vi "CAN_initialize.vi"() -> (0 "Array 2":errorcluster[](array[cluster]), 1 "Array":refnum<class "sbCANopenBaseClass.lvclass">[](array[class]), 2 "Motors to use":bool[](array[boolean]))   [LabVIEW 2017]
uses:
  <vilib>/addons/Maxon Motor/EPOS2 CANopen/CANopen/sbCANopenBaseClass.lvclass
  <vilib>/addons/Maxon Motor/EPOS2 CANopen/EPOS2 Support Files/Typedefs/EPOS2 Config Data Input Current.ctl
  <vilib>/addons/Maxon Motor/EPOS2 CANopen/EPOS2 Support Files/Typedefs/EPOS2 Velocity Units.ctl
  <vilib>/addons/Maxon Motor/EPOS2 CANopen/EPOS2 Support Files/Polymorphic SubVIs/Config/EPOS2 Current Mode Configure.vi
  <vilib>/imath/engines/lvmath2/RunTimeEngine/BuiltInFunctions/length/NIMS_length(GV).vi
  <instcachedir>/0/NIMS_length(GV)_08A3D13377FD4E4B96F5795FBF3698FA.lvgen/NIMS_length(GV)_08A3D13377FD4E4B96F5795FBF3698FA_003.vi
  <vilib>/imath/engines/lvmath2/RunTimeEngine/RangeToken/NIMS_Range_R2 - Integer.vi
  <instcachedir>/0/NIMS_Range_R2 - Integer_B2C3C6B11D0E4F789E1772ACB483EB02.lvgen/NIMS_Range_R2 - Integer_B2C3C6B11D0E4F789E1772ACB483EB02_000.vi
  <vilib>/imath/engines/lvmath2/RunTimeEngine/CommandStatement/MC_CommandStatement_break.vi
  <vilib>/imath/engines/lvmath2/RunTimeEngine/IndexRead/NIMS V(S).vi
  <instcachedir>/0/NIMS V(S)_0488751826AF41519A22953C041130DC.lvgen/NIMS V(S)_0488751826AF41519A22953C041130DC_003.vi
  <vilib>/imathl/engines/lvmath/Functions/Error Handling/Create Error.vi
  <vilib>/imath/engines/lvmath2/RunTimeEngine/VariableToken/NIMS_VariableToken_CondDefinedDefinedByReplace.vi
  <instcachedir>/0/NIMS_VariableToken_CondDefinedDefinedByReplace_D162CFFC24174562A9FEA619A91E1A56.lvgen/NIMS_VariableToken_CondDefinedDefinedByReplace_D162CFFC24174562A9FEA619A91E1A56_003.vi
  <vilib>/imath/engines/lvmath2/RunTimeEngine/IndexReplace/NIMS V(S)=S.vi
  <instcachedir>/0/NIMS V(S)=S_3F4D177D41884A9C969E5FA0B22E4B28.lvgen/NIMS V(S)=S_3F4D177D41884A9C969E5FA0B22E4B28_003.vi
  <vilib>/imath/engines/lvmath2/RunTimeEngine/VariableToken/NIMS_VariableToken_CondDefined.vi
  <instcachedir>/0/NIMS_VariableToken_CondDefined_6E7F1EE7F80E48298C84CF05BD736261.lvgen/NIMS_VariableToken_CondDefined_6E7F1EE7F80E48298C84CF05BD736261_004.vi
  <vilib>/imath/engines/lvmath2/RunTimeEngine/NodeEndStatement/NIMS_NodeEndStatement_Output.vi
  <instcachedir>/0/NIMS_NodeEndStatement_Output_53EC0D466D134D7ABD903AC30B43404B.lvgen/NIMS_NodeEndStatement_Output_53EC0D466D134D7ABD903AC30B43404B_004.vi
  <vilib>/imath/engines/lvmath2/RunTimeEngine/ErrorHandling/NIMS_Finalize Error.vi
  <vilib>/addons/Maxon Motor/EPOS2 CANopen/EPOS2 Library.lvlib
  <vilib>/addons/Maxon Motor/EPOS2 CANopen/CANopen/CANopen IndCom Interface/sdCANopenIndCom.lvclass
panel:
  out "size(s)":i32
  out "size(s) 2":i32
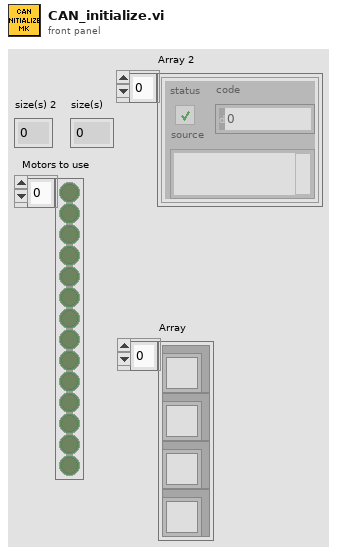
[diagram p1: front panel]
types:
  T1 = typedef "EPOS2 Library.lvlib/EPOS2 Config Data Input Current.ctl" = cluster{"Velocity Units":T2, "Max Velocity":i32}
  T2 = typedef "EPOS2 Library.lvlib/EPOS2 Velocity Units.ctl" = i8
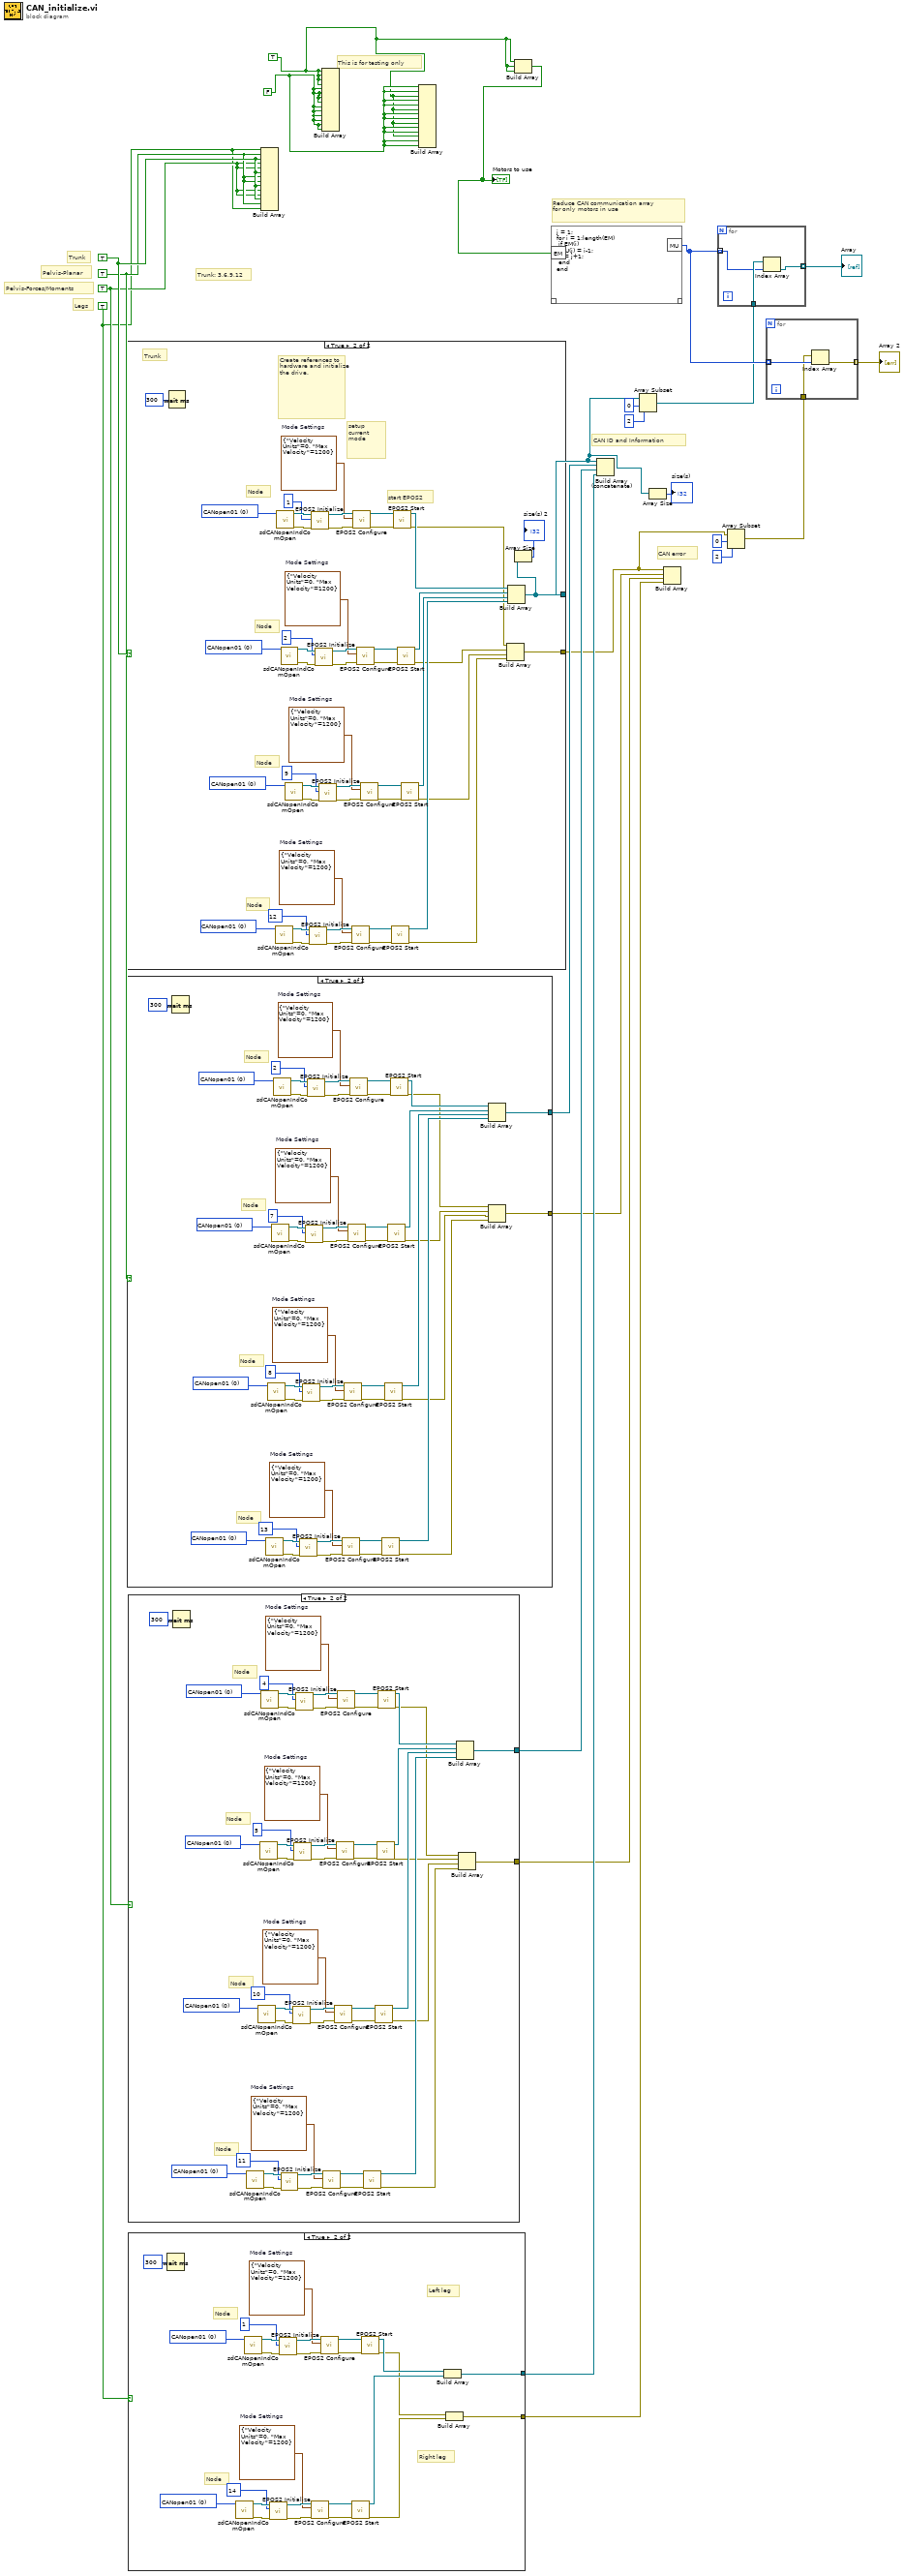
[diagram p0: block diagram]
diagram:
  w12 = FALSE
  w6 = TRUE
  w22 = TRUE
  w23 = TRUE
  w24 = TRUE
  w25 = TRUE
  # "This is for testing only"
  # "Trunk: 3,6,9,12"
  # "CAN error"
  # "CAN ID and Information"
  # "Reduce CAN communication array \nfor only motors in use"
  # "Legs"
  # "Pelvis-Forces/Moments"
  # "Pelvis-Planar"
  # "Trunk"
  n1 = case shown="True" w25 {
    tunnel: [_ w32] -> w11
    tunnel: [_ w33] -> w3
    frame False {
    }
    frame True {
      w43 = u32 0 items=["CANopen01", "CANopen02", "CANopen03", "CANopen04", "CANopen05", "CANopen06", "CANopen07", "CANopen08", "CANopen09", "CANopen10", "CANopen11", "CANopen12", "CANopen13", "CANopen14", "CANopen15", "CANopen16", "CANopen17", "CANopen18", "CANopen19", "CANopen20", "CANopen21", "CANopen22", "CANopen23", "CANopen24", "CANopen25", "CANopen26", "CANopen27", "CANopen28", "CANopen29", "CANopen30", "CANopen31", "CANopen32"] ("Interface Name")
      w44 = T1 {"Velocity Units"=0, "Max Velocity"=1200}  # Mode Settings
      w51 = u32 0 items=["CANopen01", "CANopen02", "CANopen03", "CANopen04", "CANopen05", "CANopen06", "CANopen07", "CANopen08", "CANopen09", "CANopen10", "CANopen11", "CANopen12", "CANopen13", "CANopen14", "CANopen15", "CANopen16", "CANopen17", "CANopen18", "CANopen19", "CANopen20", "CANopen21", "CANopen22", "CANopen23", "CANopen24", "CANopen25", "CANopen26", "CANopen27", "CANopen28", "CANopen29", "CANopen30", "CANopen31", "CANopen32"] ("Interface Name")
      w52 = T1 {"Velocity Units"=0, "Max Velocity"=1200}  # Mode Settings
      w59 = u32 0 items=["CANopen01", "CANopen02", "CANopen03", "CANopen04", "CANopen05", "CANopen06", "CANopen07", "CANopen08", "CANopen09", "CANopen10", "CANopen11", "CANopen12", "CANopen13", "CANopen14", "CANopen15", "CANopen16", "CANopen17", "CANopen18", "CANopen19", "CANopen20", "CANopen21", "CANopen22", "CANopen23", "CANopen24", "CANopen25", "CANopen26", "CANopen27", "CANopen28", "CANopen29", "CANopen30", "CANopen31", "CANopen32"] ("Interface Name")
      w60 = T1 {"Velocity Units"=0, "Max Velocity"=1200}  # Mode Settings
      w67 = u32 0 items=["CANopen01", "CANopen02", "CANopen03", "CANopen04", "CANopen05", "CANopen06", "CANopen07", "CANopen08", "CANopen09", "CANopen10", "CANopen11", "CANopen12", "CANopen13", "CANopen14", "CANopen15", "CANopen16", "CANopen17", "CANopen18", "CANopen19", "CANopen20", "CANopen21", "CANopen22", "CANopen23", "CANopen24", "CANopen25", "CANopen26", "CANopen27", "CANopen28", "CANopen29", "CANopen30", "CANopen31", "CANopen32"] ("Interface Name")
      w68 = T1 {"Velocity Units"=0, "Max Velocity"=1200}  # Mode Settings
      # "Node"
      # "Node"
      # "Node"
      # "Node"
      # "Trunk"
      # "Create references to hardware and initialize the drive."
      # "start EPOS2"
      # "setup current mode"
      n2 = Wait (ms)(milliseconds to wait=u32 300) -> ()  [unwired: 1 out]
      n3 = call <vilib>:"sdCANopenIndComOpen.vi"("Interface Name"=w43) -> ("error out"=w48:errorcluster, "SD CANopen Comm out"=w42:refnum<class "sbCANopenBaseClass.lvclass">)  [unwired: 9 in]
      n4 = call <vilib>:"sdCANopenIndComOpen.vi"("Interface Name"=w67) -> ("error out"=w72:errorcluster, "SD CANopen Comm out"=w66:refnum<class "sbCANopenBaseClass.lvclass">)  [unwired: 9 in]
      n5 = call <vilib>:"sdCANopenIndComOpen.vi"("Interface Name"=w59) -> ("error out"=w64:errorcluster, "SD CANopen Comm out"=w58:refnum<class "sbCANopenBaseClass.lvclass">)  [unwired: 9 in]
      n6 = call <vilib>:"sdCANopenIndComOpen.vi"("Interface Name"=w51) -> ("error out"=w56:errorcluster, "SD CANopen Comm out"=w50:refnum<class "sbCANopenBaseClass.lvclass">)  [unwired: 9 in]
      n7 = call <vilib>:"EPOS2 Initialize.vi"("error in"=w48, "Node ID"=u8 12, "CAN Session In"=w42) -> ("error out"=w49:errorcluster, "CANopen Session Out"=w46:refnum<class "sbCANopenBaseClass.lvclass">)  [unwired: 1 in, 6 out]
      n8 = call <vilib>:"EPOS2 Initialize.vi"("error in"=w72, "Node ID"=u8 1, "CAN Session In"=w66) -> ("error out"=w73:errorcluster, "CANopen Session Out"=w70:refnum<class "sbCANopenBaseClass.lvclass">)  [unwired: 1 in, 6 out]
      n9 = call <vilib>:"EPOS2 Initialize.vi"("error in"=w64, "Node ID"=u8 2, "CAN Session In"=w58) -> ("error out"=w65:errorcluster, "CANopen Session Out"=w62:refnum<class "sbCANopenBaseClass.lvclass">)  [unwired: 1 in, 6 out]
      n10 = call <vilib>:"EPOS2 Initialize.vi"("error in"=w56, "Node ID"=u8 9, "CAN Session In"=w50) -> ("error out"=w57:errorcluster, "CANopen Session Out"=w54:refnum<class "sbCANopenBaseClass.lvclass">)  [unwired: 1 in, 6 out]
      n11 = call-poly <vilib>:"EPOS2 Configure.vi"("error in"=w49, "Mode Settings"=w44, "CANopen Session In"=w46) -> ("error out"=w47:errorcluster, "CANopen Session Out"=w45:refnum<class "sbCANopenBaseClass.lvclass">)  [unwired: 7 in]
      n12 = call-poly <vilib>:"EPOS2 Configure.vi"("error in"=w73, "Mode Settings"=w68, "CANopen Session In"=w70) -> ("error out"=w71:errorcluster, "CANopen Session Out"=w69:refnum<class "sbCANopenBaseClass.lvclass">)  [unwired: 7 in]
      n13 = call-poly <vilib>:"EPOS2 Configure.vi"("error in"=w65, "Mode Settings"=w60, "CANopen Session In"=w62) -> ("error out"=w63:errorcluster, "CANopen Session Out"=w61:refnum<class "sbCANopenBaseClass.lvclass">)  [unwired: 7 in]
      n14 = call-poly <vilib>:"EPOS2 Configure.vi"("error in"=w57, "Mode Settings"=w52, "CANopen Session In"=w54) -> ("error out"=w55:errorcluster, "CANopen Session Out"=w53:refnum<class "sbCANopenBaseClass.lvclass">)  [unwired: 7 in]
      n15 = call <vilib>:"EPOS2 Start.vi"("error in"=w47, "CANopen Session In"=w45) -> ("error out"=w34:errorcluster, "CANopen Session Out"=w38:refnum<class "sbCANopenBaseClass.lvclass">)  [unwired: 8 in]
      n16 = call <vilib>:"EPOS2 Start.vi"("error in"=w71, "CANopen Session In"=w69) -> ("error out"=w37:errorcluster, "CANopen Session Out"=w41:refnum<class "sbCANopenBaseClass.lvclass">)  [unwired: 8 in]
      n17 = call <vilib>:"EPOS2 Start.vi"("error in"=w63, "CANopen Session In"=w61) -> ("error out"=w36:errorcluster, "CANopen Session Out"=w40:refnum<class "sbCANopenBaseClass.lvclass">)  [unwired: 8 in]
      n18 = call <vilib>:"EPOS2 Start.vi"("error in"=w55, "CANopen Session In"=w53) -> ("error out"=w35:errorcluster, "CANopen Session Out"=w39:refnum<class "sbCANopenBaseClass.lvclass">)  [unwired: 8 in]
      n19 = Build Array(w37, w36, w35, w34) -> (w33:errorcluster[])
      n20 = Build Array(w41, w40, w39, w38) -> (w32:refnum<class "sbCANopenBaseClass.lvclass">[])
      n21 = Array Size(array=w32) -> (size(s)=→"size(s) 2":i32)
    }
  }
  n22 = case shown="True" w24 {
    tunnel: [_ w84] -> w21
    tunnel: [_ w79] -> w17
    frame False {
    }
    frame True {
      w90 = u32 0 items=["CANopen01", "CANopen02", "CANopen03", "CANopen04", "CANopen05", "CANopen06", "CANopen07", "CANopen08", "CANopen09", "CANopen10", "CANopen11", "CANopen12", "CANopen13", "CANopen14", "CANopen15", "CANopen16", "CANopen17", "CANopen18", "CANopen19", "CANopen20", "CANopen21", "CANopen22", "CANopen23", "CANopen24", "CANopen25", "CANopen26", "CANopen27", "CANopen28", "CANopen29", "CANopen30", "CANopen31", "CANopen32"] ("Interface Name")
      w91 = T1 {"Velocity Units"=0, "Max Velocity"=1200}  # Mode Settings
      w98 = u32 0 items=["CANopen01", "CANopen02", "CANopen03", "CANopen04", "CANopen05", "CANopen06", "CANopen07", "CANopen08", "CANopen09", "CANopen10", "CANopen11", "CANopen12", "CANopen13", "CANopen14", "CANopen15", "CANopen16", "CANopen17", "CANopen18", "CANopen19", "CANopen20", "CANopen21", "CANopen22", "CANopen23", "CANopen24", "CANopen25", "CANopen26", "CANopen27", "CANopen28", "CANopen29", "CANopen30", "CANopen31", "CANopen32"] ("Interface Name")
      w99 = T1 {"Velocity Units"=0, "Max Velocity"=1200}  # Mode Settings
      w106 = u32 0 items=["CANopen01", "CANopen02", "CANopen03", "CANopen04", "CANopen05", "CANopen06", "CANopen07", "CANopen08", "CANopen09", "CANopen10", "CANopen11", "CANopen12", "CANopen13", "CANopen14", "CANopen15", "CANopen16", "CANopen17", "CANopen18", "CANopen19", "CANopen20", "CANopen21", "CANopen22", "CANopen23", "CANopen24", "CANopen25", "CANopen26", "CANopen27", "CANopen28", "CANopen29", "CANopen30", "CANopen31", "CANopen32"] ("Interface Name")
      w107 = T1 {"Velocity Units"=0, "Max Velocity"=1200}  # Mode Settings
      w114 = u32 0 items=["CANopen01", "CANopen02", "CANopen03", "CANopen04", "CANopen05", "CANopen06", "CANopen07", "CANopen08", "CANopen09", "CANopen10", "CANopen11", "CANopen12", "CANopen13", "CANopen14", "CANopen15", "CANopen16", "CANopen17", "CANopen18", "CANopen19", "CANopen20", "CANopen21", "CANopen22", "CANopen23", "CANopen24", "CANopen25", "CANopen26", "CANopen27", "CANopen28", "CANopen29", "CANopen30", "CANopen31", "CANopen32"] ("Interface Name")
      w115 = T1 {"Velocity Units"=0, "Max Velocity"=1200}  # Mode Settings
      # "Node"
      # "Node"
      # "Node"
      # "Node"
      n23 = Wait (ms)(milliseconds to wait=u32 300) -> ()  [unwired: 1 out]
      n24 = call <vilib>:"sdCANopenIndComOpen.vi"("Interface Name"=w90) -> ("error out"=w95:errorcluster, "SD CANopen Comm out"=w89:refnum<class "sbCANopenBaseClass.lvclass">)  [unwired: 9 in]
      n25 = call <vilib>:"sdCANopenIndComOpen.vi"("Interface Name"=w98) -> ("error out"=w103:errorcluster, "SD CANopen Comm out"=w97:refnum<class "sbCANopenBaseClass.lvclass">)  [unwired: 9 in]
      n26 = call <vilib>:"sdCANopenIndComOpen.vi"("Interface Name"=w106) -> ("error out"=w111:errorcluster, "SD CANopen Comm out"=w105:refnum<class "sbCANopenBaseClass.lvclass">)  [unwired: 9 in]
      n27 = call <vilib>:"sdCANopenIndComOpen.vi"("Interface Name"=w114) -> ("error out"=w119:errorcluster, "SD CANopen Comm out"=w113:refnum<class "sbCANopenBaseClass.lvclass">)  [unwired: 9 in]
      n28 = call <vilib>:"EPOS2 Initialize.vi"("error in"=w95, "Node ID"=u8 13, "CAN Session In"=w89) -> ("error out"=w96:errorcluster, "CANopen Session Out"=w93:refnum<class "sbCANopenBaseClass.lvclass">)  [unwired: 1 in, 6 out]
      n29 = call <vilib>:"EPOS2 Initialize.vi"("error in"=w103, "Node ID"=u8 8, "CAN Session In"=w97) -> ("error out"=w104:errorcluster, "CANopen Session Out"=w101:refnum<class "sbCANopenBaseClass.lvclass">)  [unwired: 1 in, 6 out]
      n30 = call <vilib>:"EPOS2 Initialize.vi"("error in"=w111, "Node ID"=u8 7, "CAN Session In"=w105) -> ("error out"=w112:errorcluster, "CANopen Session Out"=w109:refnum<class "sbCANopenBaseClass.lvclass">)  [unwired: 1 in, 6 out]
      n31 = call <vilib>:"EPOS2 Initialize.vi"("error in"=w119, "Node ID"=u8 2, "CAN Session In"=w113) -> ("error out"=w120:errorcluster, "CANopen Session Out"=w117:refnum<class "sbCANopenBaseClass.lvclass">)  [unwired: 1 in, 6 out]
      n32 = call-poly <vilib>:"EPOS2 Configure.vi"("error in"=w96, "Mode Settings"=w91, "CANopen Session In"=w93) -> ("error out"=w94:errorcluster, "CANopen Session Out"=w92:refnum<class "sbCANopenBaseClass.lvclass">)  [unwired: 7 in]
      n33 = call-poly <vilib>:"EPOS2 Configure.vi"("error in"=w104, "Mode Settings"=w99, "CANopen Session In"=w101) -> ("error out"=w102:errorcluster, "CANopen Session Out"=w100:refnum<class "sbCANopenBaseClass.lvclass">)  [unwired: 7 in]
      n34 = call-poly <vilib>:"EPOS2 Configure.vi"("error in"=w112, "Mode Settings"=w107, "CANopen Session In"=w109) -> ("error out"=w110:errorcluster, "CANopen Session Out"=w108:refnum<class "sbCANopenBaseClass.lvclass">)  [unwired: 7 in]
      n35 = call-poly <vilib>:"EPOS2 Configure.vi"("error in"=w120, "Mode Settings"=w115, "CANopen Session In"=w117) -> ("error out"=w118:errorcluster, "CANopen Session Out"=w116:refnum<class "sbCANopenBaseClass.lvclass">)  [unwired: 7 in]
      n36 = call <vilib>:"EPOS2 Start.vi"("error in"=w94, "CANopen Session In"=w92) -> ("error out"=w80:errorcluster, "CANopen Session Out"=w85:refnum<class "sbCANopenBaseClass.lvclass">)  [unwired: 8 in]
      n37 = call <vilib>:"EPOS2 Start.vi"("error in"=w102, "CANopen Session In"=w100) -> ("error out"=w81:errorcluster, "CANopen Session Out"=w86:refnum<class "sbCANopenBaseClass.lvclass">)  [unwired: 8 in]
      n38 = call <vilib>:"EPOS2 Start.vi"("error in"=w110, "CANopen Session In"=w108) -> ("error out"=w82:errorcluster, "CANopen Session Out"=w87:refnum<class "sbCANopenBaseClass.lvclass">)  [unwired: 8 in]
      n39 = call <vilib>:"EPOS2 Start.vi"("error in"=w118, "CANopen Session In"=w116) -> ("error out"=w83:errorcluster, "CANopen Session Out"=w88:refnum<class "sbCANopenBaseClass.lvclass">)  [unwired: 8 in]
      n40 = Build Array(w88, w87, w86, w85) -> (w84:refnum<class "sbCANopenBaseClass.lvclass">[])
      n41 = Build Array(w83, w82, w81, w80) -> (w79:errorcluster[])
    }
  }
  n42 = case shown="True" w23 {
    tunnel: [_ w131] -> w20
    tunnel: [_ w126] -> w16
    frame False {
    }
    frame True {
      w137 = u32 0 items=["CANopen01", "CANopen02", "CANopen03", "CANopen04", "CANopen05", "CANopen06", "CANopen07", "CANopen08", "CANopen09", "CANopen10", "CANopen11", "CANopen12", "CANopen13", "CANopen14", "CANopen15", "CANopen16", "CANopen17", "CANopen18", "CANopen19", "CANopen20", "CANopen21", "CANopen22", "CANopen23", "CANopen24", "CANopen25", "CANopen26", "CANopen27", "CANopen28", "CANopen29", "CANopen30", "CANopen31", "CANopen32"] ("Interface Name")
      w138 = T1 {"Velocity Units"=0, "Max Velocity"=1200}  # Mode Settings
      w145 = u32 0 items=["CANopen01", "CANopen02", "CANopen03", "CANopen04", "CANopen05", "CANopen06", "CANopen07", "CANopen08", "CANopen09", "CANopen10", "CANopen11", "CANopen12", "CANopen13", "CANopen14", "CANopen15", "CANopen16", "CANopen17", "CANopen18", "CANopen19", "CANopen20", "CANopen21", "CANopen22", "CANopen23", "CANopen24", "CANopen25", "CANopen26", "CANopen27", "CANopen28", "CANopen29", "CANopen30", "CANopen31", "CANopen32"] ("Interface Name")
      w146 = T1 {"Velocity Units"=0, "Max Velocity"=1200}  # Mode Settings
      w153 = u32 0 items=["CANopen01", "CANopen02", "CANopen03", "CANopen04", "CANopen05", "CANopen06", "CANopen07", "CANopen08", "CANopen09", "CANopen10", "CANopen11", "CANopen12", "CANopen13", "CANopen14", "CANopen15", "CANopen16", "CANopen17", "CANopen18", "CANopen19", "CANopen20", "CANopen21", "CANopen22", "CANopen23", "CANopen24", "CANopen25", "CANopen26", "CANopen27", "CANopen28", "CANopen29", "CANopen30", "CANopen31", "CANopen32"] ("Interface Name")
      w154 = T1 {"Velocity Units"=0, "Max Velocity"=1200}  # Mode Settings
      w161 = u32 0 items=["CANopen01", "CANopen02", "CANopen03", "CANopen04", "CANopen05", "CANopen06", "CANopen07", "CANopen08", "CANopen09", "CANopen10", "CANopen11", "CANopen12", "CANopen13", "CANopen14", "CANopen15", "CANopen16", "CANopen17", "CANopen18", "CANopen19", "CANopen20", "CANopen21", "CANopen22", "CANopen23", "CANopen24", "CANopen25", "CANopen26", "CANopen27", "CANopen28", "CANopen29", "CANopen30", "CANopen31", "CANopen32"] ("Interface Name")
      w162 = T1 {"Velocity Units"=0, "Max Velocity"=1200}  # Mode Settings
      # "Node"
      # "Node"
      # "Node"
      # "Node"
      n43 = Wait (ms)(milliseconds to wait=u32 300) -> ()  [unwired: 1 out]
      n44 = call <vilib>:"sdCANopenIndComOpen.vi"("Interface Name"=w137) -> ("error out"=w142:errorcluster, "SD CANopen Comm out"=w136:refnum<class "sbCANopenBaseClass.lvclass">)  [unwired: 9 in]
      n45 = call <vilib>:"sdCANopenIndComOpen.vi"("Interface Name"=w145) -> ("error out"=w150:errorcluster, "SD CANopen Comm out"=w144:refnum<class "sbCANopenBaseClass.lvclass">)  [unwired: 9 in]
      n46 = call <vilib>:"sdCANopenIndComOpen.vi"("Interface Name"=w153) -> ("error out"=w158:errorcluster, "SD CANopen Comm out"=w152:refnum<class "sbCANopenBaseClass.lvclass">)  [unwired: 9 in]
      n47 = call <vilib>:"sdCANopenIndComOpen.vi"("Interface Name"=w161) -> ("error out"=w166:errorcluster, "SD CANopen Comm out"=w160:refnum<class "sbCANopenBaseClass.lvclass">)  [unwired: 9 in]
      n48 = call <vilib>:"EPOS2 Initialize.vi"("error in"=w142, "Node ID"=u8 11, "CAN Session In"=w136) -> ("error out"=w143:errorcluster, "CANopen Session Out"=w140:refnum<class "sbCANopenBaseClass.lvclass">)  [unwired: 1 in, 6 out]
      n49 = call <vilib>:"EPOS2 Initialize.vi"("error in"=w150, "Node ID"=u8 10, "CAN Session In"=w144) -> ("error out"=w151:errorcluster, "CANopen Session Out"=w148:refnum<class "sbCANopenBaseClass.lvclass">)  [unwired: 1 in, 6 out]
      n50 = call <vilib>:"EPOS2 Initialize.vi"("error in"=w158, "Node ID"=u8 5, "CAN Session In"=w152) -> ("error out"=w159:errorcluster, "CANopen Session Out"=w156:refnum<class "sbCANopenBaseClass.lvclass">)  [unwired: 1 in, 6 out]
      n51 = call <vilib>:"EPOS2 Initialize.vi"("error in"=w166, "Node ID"=u8 4, "CAN Session In"=w160) -> ("error out"=w167:errorcluster, "CANopen Session Out"=w164:refnum<class "sbCANopenBaseClass.lvclass">)  [unwired: 1 in, 6 out]
      n52 = call-poly <vilib>:"EPOS2 Configure.vi"("error in"=w143, "Mode Settings"=w138, "CANopen Session In"=w140) -> ("error out"=w141:errorcluster, "CANopen Session Out"=w139:refnum<class "sbCANopenBaseClass.lvclass">)  [unwired: 7 in]
      n53 = call-poly <vilib>:"EPOS2 Configure.vi"("error in"=w151, "Mode Settings"=w146, "CANopen Session In"=w148) -> ("error out"=w149:errorcluster, "CANopen Session Out"=w147:refnum<class "sbCANopenBaseClass.lvclass">)  [unwired: 7 in]
      n54 = call-poly <vilib>:"EPOS2 Configure.vi"("error in"=w159, "Mode Settings"=w154, "CANopen Session In"=w156) -> ("error out"=w157:errorcluster, "CANopen Session Out"=w155:refnum<class "sbCANopenBaseClass.lvclass">)  [unwired: 7 in]
      n55 = call-poly <vilib>:"EPOS2 Configure.vi"("error in"=w167, "Mode Settings"=w162, "CANopen Session In"=w164) -> ("error out"=w165:errorcluster, "CANopen Session Out"=w163:refnum<class "sbCANopenBaseClass.lvclass">)  [unwired: 7 in]
      n56 = call <vilib>:"EPOS2 Start.vi"("error in"=w141, "CANopen Session In"=w139) -> ("error out"=w127:errorcluster, "CANopen Session Out"=w132:refnum<class "sbCANopenBaseClass.lvclass">)  [unwired: 8 in]
      n57 = call <vilib>:"EPOS2 Start.vi"("error in"=w149, "CANopen Session In"=w147) -> ("error out"=w128:errorcluster, "CANopen Session Out"=w133:refnum<class "sbCANopenBaseClass.lvclass">)  [unwired: 8 in]
      n58 = call <vilib>:"EPOS2 Start.vi"("error in"=w157, "CANopen Session In"=w155) -> ("error out"=w129:errorcluster, "CANopen Session Out"=w134:refnum<class "sbCANopenBaseClass.lvclass">)  [unwired: 8 in]
      n59 = call <vilib>:"EPOS2 Start.vi"("error in"=w165, "CANopen Session In"=w163) -> ("error out"=w130:errorcluster, "CANopen Session Out"=w135:refnum<class "sbCANopenBaseClass.lvclass">)  [unwired: 8 in]
      n60 = Build Array(w135, w134, w133, w132) -> (w131:refnum<class "sbCANopenBaseClass.lvclass">[])
      n61 = Build Array(w130, w129, w128, w127) -> (w126:errorcluster[])
    }
  }
  n62 = case shown="True" w22 {
    tunnel: [_ w174] -> w19
    tunnel: [_ w171] -> w15
    frame False {
    }
    frame True {
      w178 = u32 0 items=["CANopen01", "CANopen02", "CANopen03", "CANopen04", "CANopen05", "CANopen06", "CANopen07", "CANopen08", "CANopen09", "CANopen10", "CANopen11", "CANopen12", "CANopen13", "CANopen14", "CANopen15", "CANopen16", "CANopen17", "CANopen18", "CANopen19", "CANopen20", "CANopen21", "CANopen22", "CANopen23", "CANopen24", "CANopen25", "CANopen26", "CANopen27", "CANopen28", "CANopen29", "CANopen30", "CANopen31", "CANopen32"] ("Interface Name")
      w179 = T1 {"Velocity Units"=0, "Max Velocity"=1200}  # Mode Settings
      w186 = u32 0 items=["CANopen01", "CANopen02", "CANopen03", "CANopen04", "CANopen05", "CANopen06", "CANopen07", "CANopen08", "CANopen09", "CANopen10", "CANopen11", "CANopen12", "CANopen13", "CANopen14", "CANopen15", "CANopen16", "CANopen17", "CANopen18", "CANopen19", "CANopen20", "CANopen21", "CANopen22", "CANopen23", "CANopen24", "CANopen25", "CANopen26", "CANopen27", "CANopen28", "CANopen29", "CANopen30", "CANopen31", "CANopen32"] ("Interface Name")
      w187 = T1 {"Velocity Units"=0, "Max Velocity"=1200}  # Mode Settings
      # "Right leg"
      # "Left leg"
      # "Node"
      # "Node"
      n63 = Wait (ms)(milliseconds to wait=u32 300) -> ()  [unwired: 1 out]
      n64 = call <vilib>:"sdCANopenIndComOpen.vi"("Interface Name"=w178) -> ("error out"=w183:errorcluster, "SD CANopen Comm out"=w177:refnum<class "sbCANopenBaseClass.lvclass">)  [unwired: 9 in]
      n65 = call <vilib>:"sdCANopenIndComOpen.vi"("Interface Name"=w186) -> ("error out"=w191:errorcluster, "SD CANopen Comm out"=w185:refnum<class "sbCANopenBaseClass.lvclass">)  [unwired: 9 in]
      n66 = call <vilib>:"EPOS2 Initialize.vi"("error in"=w183, "Node ID"=u8 14, "CAN Session In"=w177) -> ("error out"=w184:errorcluster, "CANopen Session Out"=w181:refnum<class "sbCANopenBaseClass.lvclass">)  [unwired: 1 in, 6 out]
      n67 = call <vilib>:"EPOS2 Initialize.vi"("error in"=w191, "Node ID"=u8 1, "CAN Session In"=w185) -> ("error out"=w192:errorcluster, "CANopen Session Out"=w189:refnum<class "sbCANopenBaseClass.lvclass">)  [unwired: 1 in, 6 out]
      n68 = call-poly <vilib>:"EPOS2 Configure.vi"("error in"=w184, "Mode Settings"=w179, "CANopen Session In"=w181) -> ("error out"=w182:errorcluster, "CANopen Session Out"=w180:refnum<class "sbCANopenBaseClass.lvclass">)  [unwired: 7 in]
      n69 = call-poly <vilib>:"EPOS2 Configure.vi"("error in"=w192, "Mode Settings"=w187, "CANopen Session In"=w189) -> ("error out"=w190:errorcluster, "CANopen Session Out"=w188:refnum<class "sbCANopenBaseClass.lvclass">)  [unwired: 7 in]
      n70 = call <vilib>:"EPOS2 Start.vi"("error in"=w182, "CANopen Session In"=w180) -> ("error out"=w172:errorcluster, "CANopen Session Out"=w175:refnum<class "sbCANopenBaseClass.lvclass">)  [unwired: 8 in]
      n71 = call <vilib>:"EPOS2 Start.vi"("error in"=w190, "CANopen Session In"=w188) -> ("error out"=w173:errorcluster, "CANopen Session Out"=w176:refnum<class "sbCANopenBaseClass.lvclass">)  [unwired: 8 in]
      n72 = Build Array(w176, w175) -> (w174:refnum<class "sbCANopenBaseClass.lvclass">[])
      n73 = Build Array(w173, w172) -> (w171:errorcluster[])
    }
  }
  n74 = Build Array(w22, w24, w25, w23, w23, w25, w24, w24, w25, w23, w23, w25, w24, w22) -> ()  [unwired: 1 out]
  n75 = Build Array(w6, w6, w6, w6, w12, w12, w12, w12, w12, w12, w12, w12, w12, w12) -> ()  [unwired: 1 out]
  n76 = Build Array(w12, w12, w6, w12, w12, w6, w12, w12, w6, w12, w12, w6, w12, w12) -> ()  [unwired: 1 out]
  n77 = Build Array(w6, w6, w6) -> (w7:bool[])
  "Motors to use" <- w7
  n78 = mathscript code="j = 1;\nfor i = 1:length(EM)\n if EM(i)\n  MU(j) = i-1;\n  j = j+1;\n end\nend"("EM"=w7) -> ("MU"=w18:i32[])  [unwired: 1 in, 1 out]
  n79 = Build Array (concatenate)(w11, w21, w20, w19) -> ()  [unwired: 1 out]
  n80 = Array Subset(array=w11, index=0, length=2) -> (w8:refnum<class "sbCANopenBaseClass.lvclass">[])
  n81 = Array Size(array=w11) -> (size(s)=→"size(s)":i32)
  n82 = Build Array(w3, w17, w16, w15) -> ()  [unwired: 1 out]
  n83 = for {
    tunnel: w18 -> [w194] mode=indexing
    tunnel: w8 -> [w195]
    tunnel: [w193] -> w13 mode=indexing
    n84 = Index Array(array=w195, index=w194) -> (element=w193:refnum<class "sbCANopenBaseClass.lvclass">)
  }
  "Array" <- w13
  n85 = Array Subset(array=w3, index=0, length=2) -> (w2:errorcluster[])
  n86 = for {
    tunnel: [w198] -> w1 mode=indexing
    tunnel: w18 -> [w197] mode=indexing
    tunnel: w2 -> [w196]
    n87 = Index Array(array=w196, index=w197) -> (element=w198:errorcluster)
  }
  "Array 2" <- w1
